vi "Elevator Controller.vi"(8 "error in":errorcluster) -> ()   [LabVIEW 2018]
doc: "This VI executes continuously carrying out the current operation and responding to updates or new operations. It will often contain the timing or control code that is difficult to place directly in TeleOp. This VI generally opens all sensors and motors and isolates the rest of the robot code from knowing how the operations are carried out."
uses:
  <vilib>/Rock Robotics/WPI/Framework/Completion Status.ctl
  Elevator Setpoints.ctl
  Elevator Operations.ctl
  Infrastructure/Positions.ctl
  <vilib>/Rock Robotics/WPI/ThirdParty/REV Robotics/SPARK MAX/Typedef/Spark MAX Idle Mode.ctl
  <vilib>/Rock Robotics/WPI/ThirdParty/REV Robotics/SPARK MAX/Typedef/Spark MAX Control Type.ctl
  <vilib>/Rock Robotics/Network Tables/NT Read String.vi
  <vilib>/Rock Robotics/Network Tables/NT Write Number.vi
  Framework/Robot Global Data.vi
panel:
  in  "Interactive Values":T1={"Operation"=enum."Reserve", "Manual Input"=0.0, "Position"=enum."Bottom Pannel", "1/3 Power"=FALSE}
  out "Current\nCmd":string
  in  "Buttons":cluster{"Execute Cmd":bool, "Abort Cmd":bool}
  out "Command Timing":cluster{"Start Time (ms)":u32, "Iterations":i32}
  out "Status":T4
  # "Interactive Command: You may fill in the settings for a command\nand schedule it with the Execute button. You can observe and abort\nany command while fine tuning the code for the controller."
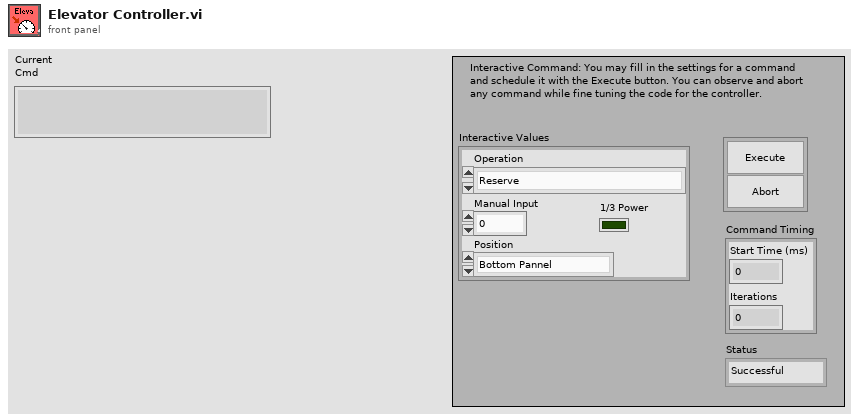
[diagram p1: front panel]
types:
  T1 = typedef "Elevator Setpoints.ctl" = cluster{"Operation":T2, "Manual Input":dbl, "Position":T3, "1/3 Power":bool}
  T2 = typedef "Elevator Operations.ctl" = enum16{"Reserve", "Read Current", "Immediate"}
  T3 = typedef "Positions.ctl" = enum16{"MANUAL", "Bottom Pannel", "Bottom Cargo", "Feeder Station", "Cargo Ship Cargo", "Middle Pannel", "Middle Cargo", "Top Pannel", "Top Cargo"}
  T4 = typedef "Completion Status.ctl" = enum16{"Successful", "Aborted", "Incomplete"}
  T5 = typedef "Spark MAX Idle Mode.ctl" = enum16{"Coast", "Brake"}
  T6 = typedef "WPI_MotorControlDeviceRef.ctl" = cluster{"DeviceStatus":errorcluster, "Type":T7, "PWM":cluster{"PWM Channel":T8, "DeadBand":T9}, "CAN":cluster{"Device Number":u8, "SetOutput VI Ref":variant, "GetOutput VI Ref":variant, "Enable VI Ref":variant, "Disable VI Ref":variant, "Data":variant}, "Invert":bool, "DIO PWM":cluster{"PWM \"Enable\" Channel":T8, "DIOChannel":T10, "PWM Rate":dbl}}
  T7 = typedef "WPI_MotorControlType.ctl" = enum16{"PWM", "CAN", "DIO PWM"}
  T8 = typedef "FPGA_DIOPWMChannel.ctl" = enum8{"PWM 0", "PWM 1", "PWM 2", "PWM 3", "PWM 4", "PWM 5", "PWM 6", "PWM 7", "PWM 8", "PWM 9", "PWM MXP 0", "PWM MXP 1", "PWM MXP 2", "PWM MXP 3", "PWM MXP 4", "PWM MXP 5", "PWM MXP 6", "PWM MXP 7", "PWM MXP 8", "PWM MXP 9", "Invalid"}
  T9 = typedef "WPI_PWMDeadband.ctl" = cluster{"Name":string, "maxPositivePwm":i32, "minPositivePwm":i32, "centerPwm":i32, "maxNegativePwm":i32, "minNegativePwm":i32, "angularRange":u16}
  T10 = typedef "FPGA_DIOChannel.ctl" = enum8{"DIO 0", "DIO 1", "DIO 2", "DIO 3", "DIO 4", "DIO 5", "DIO 6", "DIO 7", "DIO 8", "DIO 9", "DIO MXP 0", "DIO MXP 1", "DIO MXP 2", "DIO MXP 3", "DIO MXP 4", "DIO MXP 5", "DIO MXP 6", "DIO MXP 7", "DIO MXP 8", "DIO MXP 9", "DIO MXP 10", "DIO MXP 11", "DIO MXP 12", "DIO MXP 13", "DIO MXP 14", "DIO MXP 15", "SPI Port CS1", "SPI Port CS2", "SPI Port CS3", "SPI Port MISO", "SPI Port MOSI", "Invalid"}
  T11 = typedef "Command Status Info.ctl" = cluster{"Name":string, "Status":T4, "notifier out":T12}
  T12 = typedef "Completion Notifier.ctl" = refnum<notifier>
  T13 = cluster{"Current Command":T1, "Command Timing":cluster{"Start Time (ms)":u32, "Iterations":i32}, "Command Arguments":cluster{"Command Info":T11, "Description":string, "Default Command":T1, "queue out":refnum<queue>, "Subsystem Name":string}}
  T14 = cluster{"P Gain":dbl, "I Gain":dbl, "D Gain":dbl, "F Gain":dbl, "I Zone":dbl, "Min Output":dbl, "Max Output":dbl}
  T15 = typedef "Spark MAX Control Type.ctl" = enum16{"Percent VBus", "Voltage", "Velocity", "Position", "Smart Motion", "Current", "Smart Velocity"}
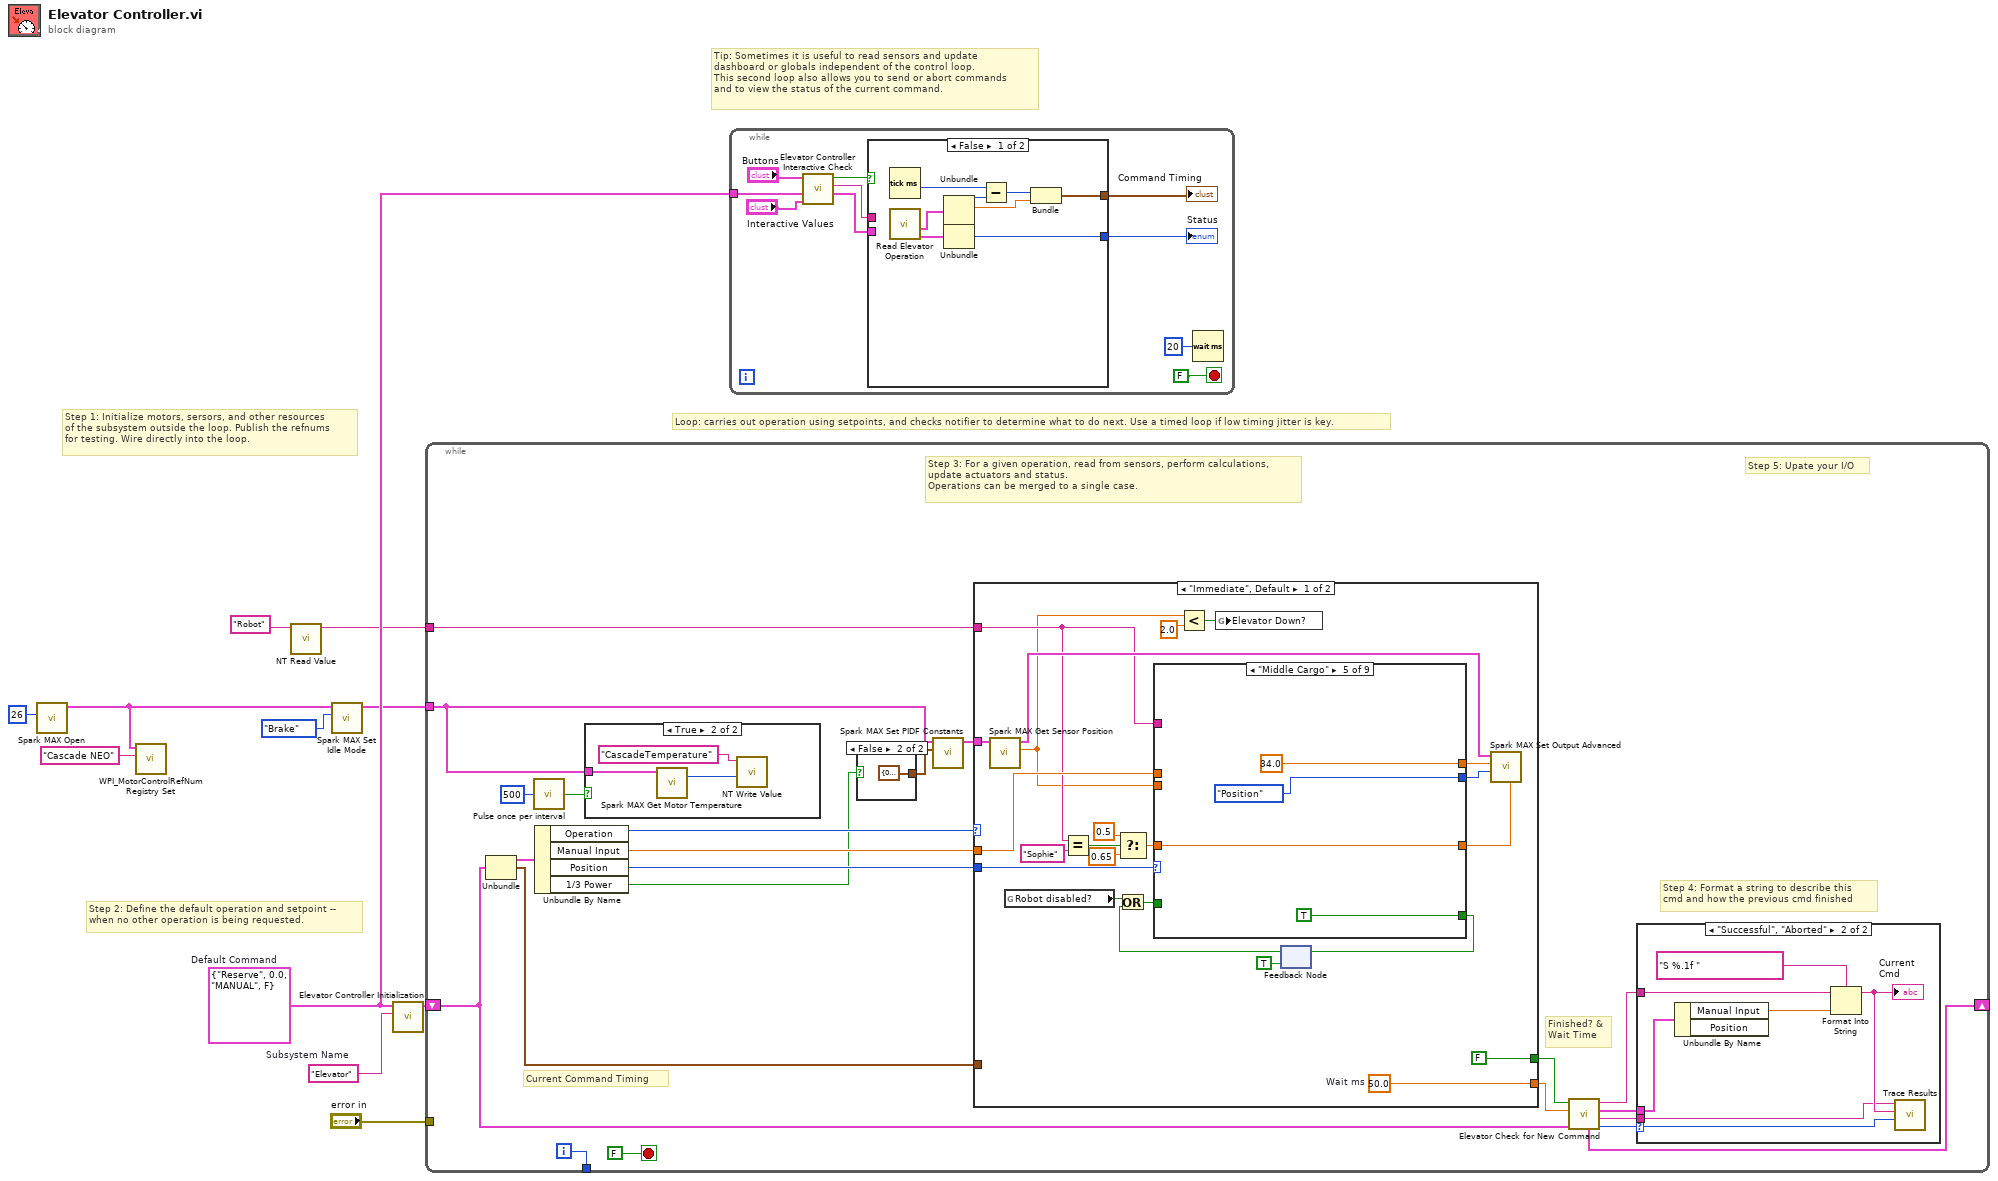
[diagram p0: block diagram]
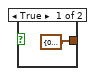
[diagram p3: hidden frame]
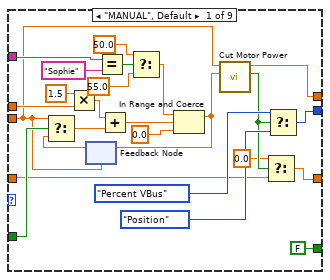
[diagram p4: hidden frame]
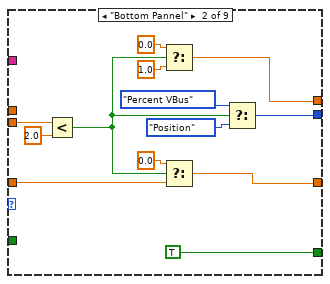
[diagram p5: hidden frame]
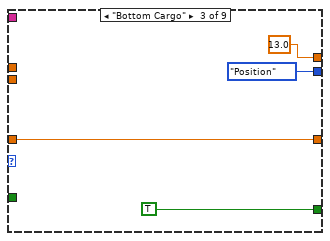
[diagram p6: hidden frame]
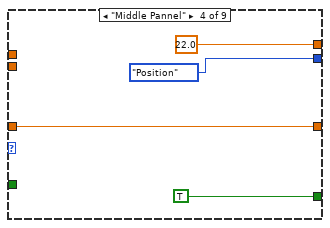
[diagram p7: hidden frame]
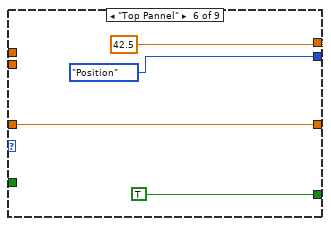
[diagram p8: hidden frame]
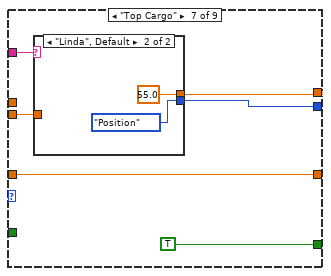
[diagram p9: hidden frame]
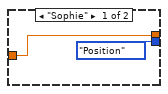
[diagram p10: hidden frame]
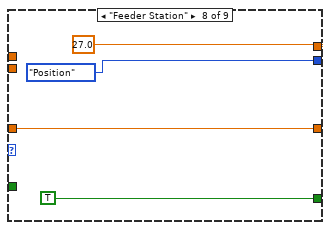
[diagram p11: hidden frame]
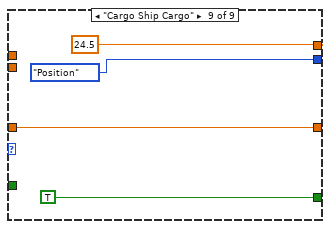
[diagram p12: hidden frame]
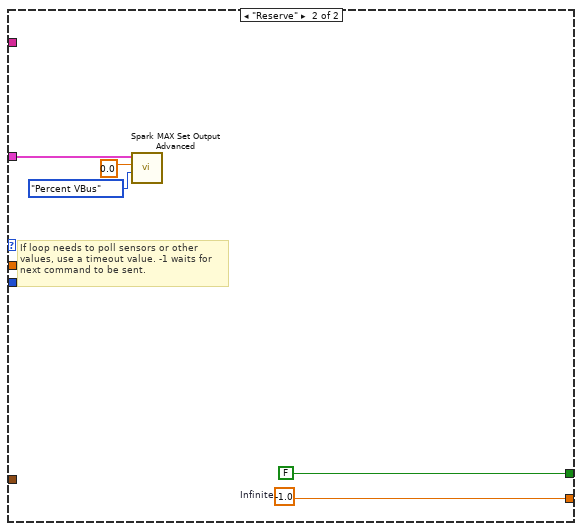
[diagram p13: hidden frame]
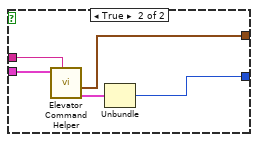
[diagram p15: hidden frame]
diagram:
  w8 = T1 {"Operation"=enum."Reserve", "Manual Input"=0.0, "Position"=enum."MANUAL", "1/3 Power"=FALSE}  # Default Command
  w9 = "Elevator"  # Subsystem Name
  # "Tip: Sometimes it is useful to read sensors and update\ndashboard or globals independent of the control loop.\nThis second loop also allows you to send or abort commands\nand to view the status of the current command."
  # "Step 2: Define the default operation and setpoint --\nwhen no other operation is being requested."
  # "Step 1: Initialize motors, sersors, and other resources\nof the subsystem outside the loop. Publish the refnums\nfor testing. Wire directly into the loop."
  # "Loop: carries out operation using setpoints, and checks notifier to determine what to do next. Use a timed loop if low timing jitter is key."
  n1 = call <vilib>:"Spark MAX Open.vi"("Device Number"=u8 26) -> ("MotorControlDeviceRef"=w2:T6)  [unwired: 9 in, 1 out]
  n2 = call <vilib>:"WPI_MotorControlRefNum Registry Set.vi"("refnum name"="Cascade NEO", "MotorControlDevRef"=w2) -> ()  [unwired: 8 in, 2 out]
  n3 = call-poly <vilib>:"NT Read Value.vi"("Name"="Robot") -> ("String"=w4:string)  [unwired: 9 in, 1 out]
  n4 = call <vilib>:"Spark MAX Set Idle Mode.vi"("Idle Mode"=Spark_MAX_Idle_Mode."Brake", "MotorControlDeviceRef in"=w2) -> ("MotorControlDeviceRef out"=w3:T6)  [unwired: 8 in, 1 out]
  n5 = call "Elevator Controller Initialization.vi"("Subsystem Name"=w9, "Default Command"=w8) -> ("Current Command"=w10:T13)  [unwired: 9 in]
  n6 = while {
    shift-right: [w27] -> _
    shift-left: w10 -> [w16]
    tunnel: [w32] -> _
    tunnel: "error in" -> [_]
    tunnel: w3 -> [w14]
    tunnel: w4 -> [w18]
    i -> [w32]
    stop <- FALSE stop-if-true
    # "Step 5: Upate your I/O"
    # "Step 4: Format a string to describe this\ncmd and how the previous cmd finished"
    # "Current Command Timing"
    # "Finished? &\nWait Time"
    # "Step 3: For a given operation, read from sensors, perform calculations,\nupdate actuators and status.\nOperations can be merged to a single case."
    n7 = Unbundle(w16) -> ("Current Command"=w31:T1, "Command Timing"=w28:cluster{"Start Time (ms)":u32, "Iterations":i32})  [unwired: 1 out]
    n8 = call "Pulse once per interval.vi"("Time (ms)"=u32 500) -> ("Boolean"=w12:bool)
    n9 = Unbundle By Name(w31) -> ("Operation"=w30:T2, "Manual Input"=w29:dbl, "Position"=w20:T3, "1/3 Power"=w15:bool)
    n10 = case shown="True" w12 {
      tunnel: w14 -> [_ w36]
      frame False {
      }
      frame True {
        n11 = call <vilib>:"Spark MAX Get Motor Temperature.vi"("MotorControlDevRef in"=w36) -> ("Motor Temperature"=w35:u8)  [unwired: 7 in, 3 out]
        n12 = call-poly <vilib>:"NT Write Value.vi"("Numeric"=w35, "Name"="CascadeTemperature") -> ()  [unwired: 9 in, 1 out]
      }
    }
    n13 = case shown="False" w15 {
      tunnel: [T14 {"P Gain"=0.05, "I Gain"=1e-05, "D Gain"=1e-05, "F Gain"=0.0, "I Zone"=0.0, "Min Output"=-0.6, "Max Output"=0.6} ("PID Constants") T14 {"P Gain"=0.05, "I Gain"=1e-05, "D Gain"=2e-05, "F Gain"=0.0, "I Zone"=0.0, "Min Output"=-1.0, "Max Output"=1.0} ("PID Constants")] -> w19
      frame True {
      }
      frame False {
      }
    }
    n14 = call <vilib>:"Spark MAX Set PIDF Constants.vi"("PID Constants"=w19, "MotorControlDeviceRef"=w14) -> ("MotorControlDeviceRef"=w17:T6)  [unwired: 8 in, 1 out]
    n15 = case shown="\"Immediate\", Default" w30 {
      tunnel: [w61 w138] -> w25
      tunnel: [FALSE ("ignore previous (F)") FALSE ("ignore previous (F)")] -> w26
      tunnel: w28 -> [_ _]
      tunnel: w29 -> [w60 _]
      tunnel: w17 -> [w53 w136]
      tunnel: w20 -> [w56 _]
      tunnel: w18 -> [w44 _]
      frame "Immediate", Default {
        w61 = 50.0  # Wait ms
        n16 = call <vilib>:"Spark MAX Get Sensor Position.vi"("MotorControlDevRef in"=w53) -> ("Sensor Position"=w39:dbl, "MotorControlDevRef out"=w48:T6)  [unwired: 7 in, 2 out]
        n17 = global read "Robot Global Data.vi" "Robot disabled?"() -> (w50:bool)
        n18 = Equal?(x=w44, y="Sophie") -> (x = y?=w45:bool)
        n19 = Select(t=0.5 ("F Term"), s=w45, f=0.65 ("F Term")) -> (s? t:f=w47:dbl)
        n20 = Less?(x=w39, y=2.0 ("x")) -> (x < y?=w41:bool)
        n21 = global write "Robot Global Data.vi" "Elevator Down?"(w41) -> ()
        n22 = feedback #1(TRUE) -> (w51:bool)
        n23 = Or(x=w50, y=w51) -> (x .or. y?=w52:bool)
        n24 = case shown="\"Middle Cargo\"" w56 {
          tunnel: w60 -> [w84 _ _ _ _ _ _ _ _]
          tunnel: w39 -> [w67 w98 _ _ _ _ w116 _ _]
          tunnel: [w69 w91 Spark_MAX_Control_Type."Position" ("Control Mode") Spark_MAX_Control_Type."Position" ("Control Mode") Spark_MAX_Control_Type."Position" ("Control Mode") Spark_MAX_Control_Type."Position" ("Control Mode") w120 Spark_MAX_Control_Type."Position" ("Control Mode") Spark_MAX_Control_Type."Position" ("Control Mode")] -> w59
          tunnel: [w71 w92 13.0 ("Setpoint") 22.0 ("Setpoint") 34.0 ("Setpoint") 42.5 ("Setpoint") w121 27.0 ("Setpoint") 24.5 ("Setpoint")] -> w49
          tunnel: [w65 w90 w100 w104 w108 w112 w118 w126 w130] -> w58
          tunnel: [FALSE TRUE TRUE TRUE TRUE TRUE TRUE TRUE TRUE] -> w55
          tunnel: w52 -> [w78 _ _ _ _ _ _ _ _]
          tunnel: w44 -> [w77 _ _ _ _ _ w117 _ _]
          tunnel: w47 -> [w63 w87 w100 w104 w108 w112 w118 w126 w130]
          frame "MANUAL", Default {
            n25 = Multiply(x=1.5, y=w84) -> (x*y=w83:dbl)
            n26 = feedback #2(w67) -> (w80:dbl)
            n27 = Select(t=w67, s=w78, f=w80) -> (s? t:f=w79:dbl)
            n28 = Equal?(x=w77, y="Sophie") -> (x = y?=w75:bool)
            n29 = Add(x=w83, y=w79) -> (x+y=w85:dbl)
            n30 = Select(t=50.0, s=w75, f=55.0) -> (s? t:f=w74:dbl)
            n31 = In Range and Coerce(upper limit=w74, x=w85, lower limit=0.0) -> (coerced(x)=w66:dbl)  [unwired: 1 out]
            n32 = feedback-in #2(w66) -> ()
            n33 = call "Cut Motor Power.vi"("f in"=w66, "Sensor Position"=w67) -> ("Boolean"=w64:bool, "f out"=w71:dbl)  [unwired: 8 in]
            n34 = Select(t=0.0, s=w64, f=w63) -> (s? t:f=w65:dbl)
            n35 = Select(t=Spark_MAX_Control_Type."Percent VBus" ("Control Mode"), s=w64, f=Spark_MAX_Control_Type."Position" ("Control Mode")) -> (s? t:f=w69:T15)
          }
          frame "Bottom Pannel" {
            n36 = Less?(x=w98, y=2.0) -> (x < y?=w88:bool)
            n37 = Select(t=0.0 ("Output"), s=w88, f=1.0 ("Output")) -> (s? t:f=w92:dbl)
            n38 = Select(t=0.0, s=w88, f=w87) -> (s? t:f=w90:dbl)
            n39 = Select(t=Spark_MAX_Control_Type."Percent VBus", s=w88, f=Spark_MAX_Control_Type."Position" ("Control Mode")) -> (s? t:f=w91:T15)
          }
          frame "Bottom Cargo" {
          }
          frame "Middle Pannel" {
          }
          frame "Middle Cargo" {
          }
          frame "Top Pannel" {
          }
          frame "Top Cargo" {
            n40 = case shown="\"Linda\", Default" w117 {
              tunnel: [w123 55.0 ("Setpoint")] -> w121
              tunnel: [Spark_MAX_Control_Type."Position" ("Control Mode") Spark_MAX_Control_Type."Position" ("Control Mode")] -> w120
              tunnel: w116 -> [w123 _]
              frame "Sophie" {
              }
              frame "Linda", Default {
              }
            }
          }
          frame "Feeder Station" {
          }
          frame "Cargo Ship Cargo" {
          }
        }
        n41 = feedback-in #1(w55) -> ()
        n42 = call <vilib>:"Spark MAX Set Output Advanced.vi"("Arbitrary Feed Forward (0)"=w58, "Control Mode"=w59, "Setpoint"=w49, "MotorControlDevRef"=w48) -> ()  [unwired: 6 in, 2 out]
      }
      frame "Reserve" {
        w138 = -1.0  # Infinite
        # "If loop needs to poll sensors or other\nvalues, use a timeout value. -1 waits for\nnext command to be sent."
        n43 = call <vilib>:"Spark MAX Set Output Advanced.vi"("Control Mode"=Spark_MAX_Control_Type."Percent VBus", "Setpoint"=0.0, "MotorControlDevRef"=w136) -> ()  [unwired: 7 in, 2 out]
      }
    }
    n44 = call "Elevator Check for New Command.vi"("Current Command"=w16, "Wait time (ms)"=w25, "Finished?"=w26) -> ("Completion"=w21:T4, "Subsystem Name"=w22:string, "Current Command"=w23:T1, "Initial Trace String"=w24:string, "NextCommand"=w27:T13)  [unwired: 4 in]
    n45 = case shown="\"Successful\", \"Aborted\"" w21 {
      selector: w21 -> [_ w145]
      tunnel: w24 -> [_ w141]
      tunnel: w23 -> [_ w142]
      tunnel: w22 -> [_ w139]
      frame "Incomplete", Default {
        # "Continuing current command"
      }
      frame "Successful", "Aborted" {
        # "Report and setup for next command"
        n46 = Unbundle By Name(w142) -> ("Manual Input"=w144:dbl)  [unwired: 1 out]
        n47 = Format Into String(format string="S %.1f ", initial string=w141, w144) -> (resulting string=w140:string)  [unwired: 1 in, 1 out]
        "Current\nCmd" <- w140
        n48 = call <vilib>:"Trace Results.vi"("Status of previous command"=w145, "Description"=w140, "Subsystem"=w139) -> ()  [unwired: 9 in]
      }
    }
  }
  n49 = while {
    tunnel: w8 -> [w152]
    stop <- FALSE stop-if-true
    n50 = call "Elevator Controller Interactive Check.vi"("Interactive Command in"="Interactive Values", "Default Command"=w152, "Buttons"="Buttons") -> ("Interactive Command out"=w149:T1, "Trace String"=w150:string, "Schedule"=w151:bool)  [unwired: 6 in]
    n51 = case shown="False" w151 {
      tunnel: [w163 w168] -> w148
      tunnel: w149 -> [_ w166]
      tunnel: [w159 w164] -> w147
      tunnel: w150 -> [_ w167]
      frame False {
        n52 = Tick Count (ms)() -> (millisecond timer value=w158:u32)
        n53 = call "Read Elevator Operation.vi"() -> ("Command Info"=w156:T11, "SubSystem Data"=w157:T1)  [unwired: 9 in, 1 out]
        n54 = Unbundle(w157) -> ("Operation"=w162:T2, "Manual Input"=w160:dbl)  [unwired: 2 out]
        n55 = Unbundle(w156) -> ("Status"=w163:T4)  [unwired: 2 out]
        n56 = Subtract(x=w158, y=w162) -> (x-y=w161:u32)
        n57 = Bundle(w161, "Manual Input"=w160) -> (w159:cluster{u32, "Manual Input":dbl})  [unwired: 1 in]
      }
      frame True {
        n58 = call "Elevator Command Helper.vi"("Description"=w167, "SubSystem Data"=w166) -> ("Command Info Out"=w165:T11, "Command Timing"=w164:cluster{"Start Time (ms)":u32, "Iterations":i32})  [unwired: 7 in, 1 out]
        n59 = Unbundle(w165) -> ("Status"=w168:T4)  [unwired: 2 out]
      }
    }
    "Status" <- w148
    "Command Timing" <- w147
    n60 = Wait (ms)(milliseconds to wait=u32 20) -> ()  [unwired: 1 out]
  }
